vi "Boolean to Boolean String.vi"(1 "Boolean":bool) -> (0 "T/F String":string)   [LabVIEW 2015, in "CS++Utilities.lvlib"]
doc: "Convert Boolean to boolean string (True or False)."
uses:
  CS++Utilities.lvlib
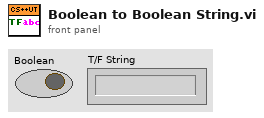
[diagram p1: front panel]
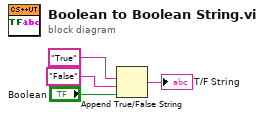
[diagram p0: block diagram]
diagram:
  n1 = Append True/False String(1:"Boolean", 2:"False" ("string"), 3:"True" ("true string")) -> (0:→"T/F String":string)  [unwired: 1 in]
